vi "质控单元流程步骤.vi"() -> ()   [LabVIEW 2016]
panel:
  out "步骤时间/秒":T1={"步骤1时间"=2, "步骤2时间"=4, "步骤3时间"=2, "步骤4时间"=5, "步骤5时间"=6, "步骤6时间"=3, "步骤7时间"=4, "步骤8时间"=7, "步骤9时间"=8, "步骤10时间"=6}
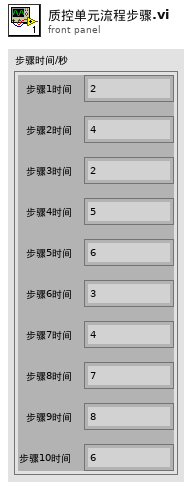
[diagram p1: front panel]
types:
  T1 = cluster{"步骤1时间":i32, "步骤2时间":i32, "步骤3时间":i32, "步骤4时间":i32, "步骤5时间":i32, "步骤6时间":i32, "步骤7时间":i32, "步骤8时间":i32, "步骤9时间":i32, "步骤10时间":i32}
  T2 = enum16{"步骤1", "步骤2", "步骤3", "步骤4", "步骤5", "步骤6", "步骤7", "步骤8", "步骤9", "步骤10"}
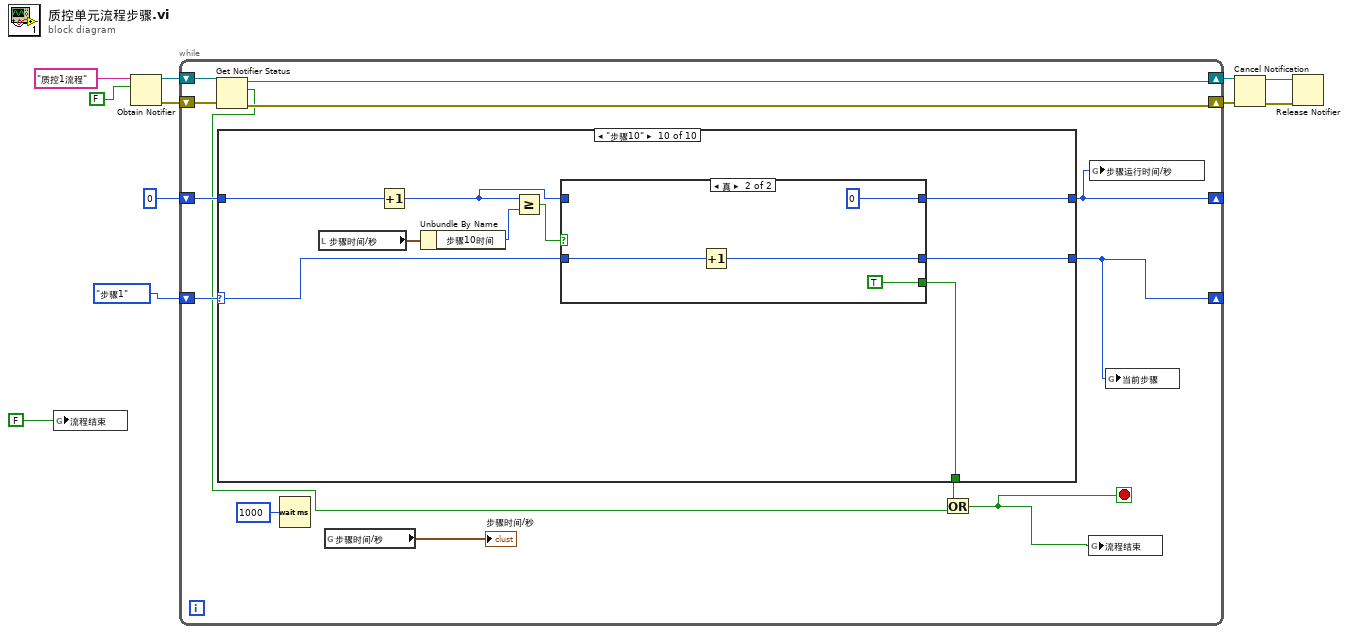
[diagram p0: block diagram]
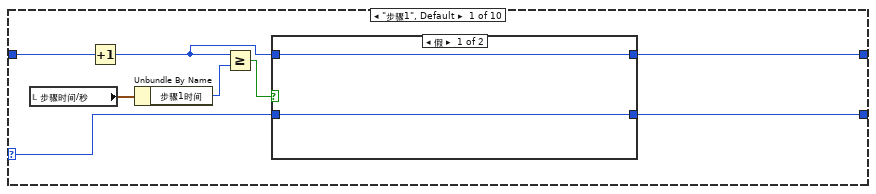
[diagram p2: hidden frame]
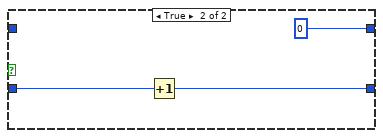
[diagram p3: hidden frame]
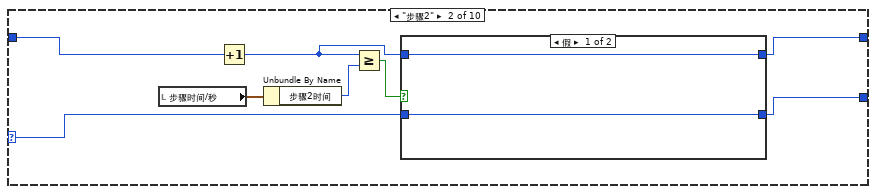
[diagram p4: hidden frame]
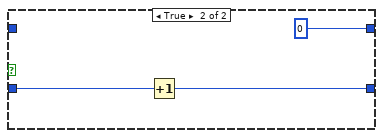
[diagram p5: hidden frame]
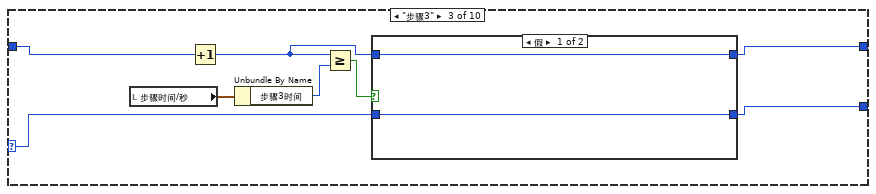
[diagram p6: hidden frame]
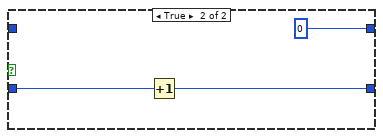
[diagram p7: hidden frame]
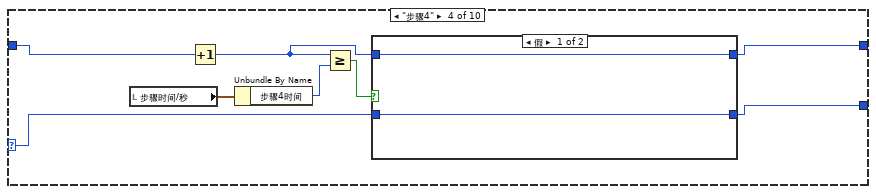
[diagram p8: hidden frame]
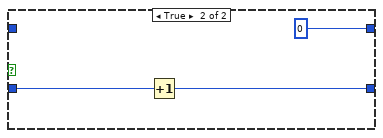
[diagram p9: hidden frame]
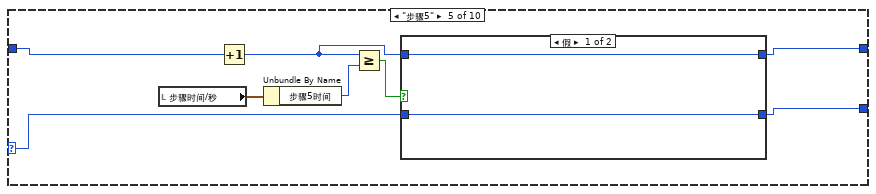
[diagram p10: hidden frame]
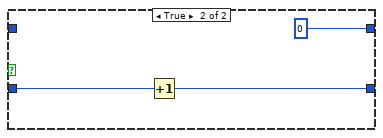
[diagram p11: hidden frame]
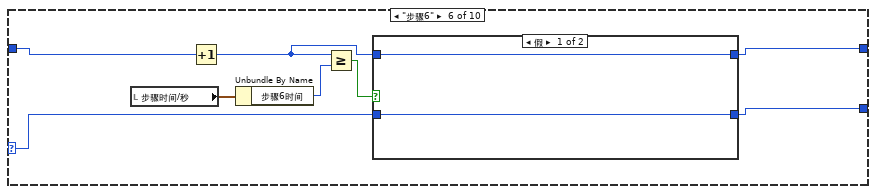
[diagram p12: hidden frame]
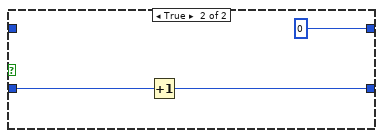
[diagram p13: hidden frame]
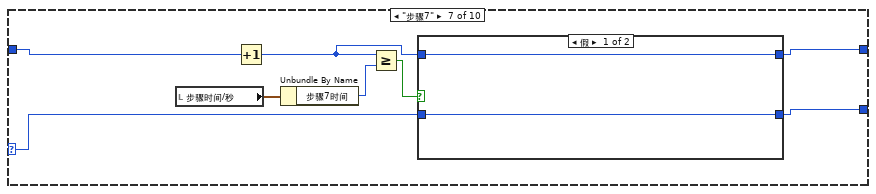
[diagram p14: hidden frame]
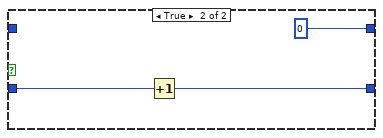
[diagram p15: hidden frame]
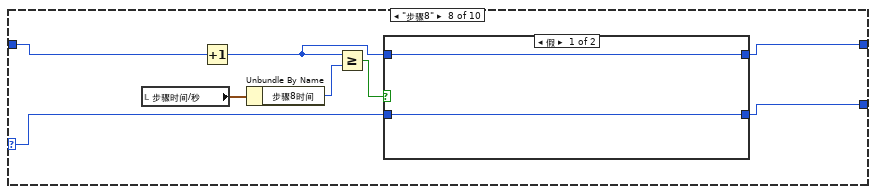
[diagram p16: hidden frame]
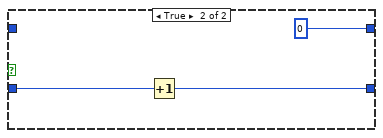
[diagram p17: hidden frame]
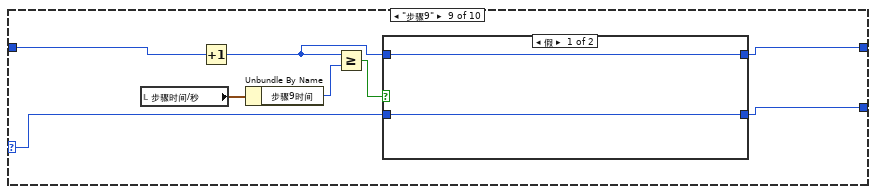
[diagram p18: hidden frame]
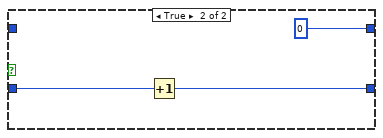
[diagram p19: hidden frame]
diagram:
  n1 = global write "质控单元全局.vi" "流程结束"(FALSE ("流程结束")) -> ()
  n2 = Obtain Notifier(name (unnamed)="质控1流程" ("名称（未命名）"), notification data type=FALSE) -> (notifier out=w7:refnum<notifier>, error out=w6:errorcluster)  [unwired: 2 in, 1 out]
  n3 = while {
    shift-right: [w13] -> _
    shift-left: T2."步骤1" -> [w24]
    shift-right: [w12] -> _
    shift-left: 0 -> [w22]
    shift-right: [w18] -> w3
    shift-left: w7 -> [w20]
    shift-right: [w17] -> w2
    shift-left: w6 -> [w19]
    stop <- w14 stop-if-true
    n4 = Get Notifier Status(notifier=w20, error in (no error)=w19) -> (notifier out=w18:refnum<notifier>, current notification=w16:bool, error out=w17:errorcluster)  [unwired: 2 out]
    n5 = case shown="\"步骤10\"" w24 {
      selector: w24 -> [w26 w40 w53 w66 w79 w92 w105 w118 w131 w145]
      tunnel: [_ _ _ _ _ _ _ _ _ w142] -> w21
      tunnel: w22 -> [w32 w41 w54 w67 w80 w93 w106 w119 w132 w146]
      tunnel: [w28 w39 w52 w65 w78 w91 w104 w117 w130 w144] -> w12
      tunnel: [w25 w38 w51 w64 w77 w90 w103 w116 w129 w143] -> w13
      frame "步骤1", Default {
        n6 = local read "步骤时间/秒"() -> (w31:T1)
        n7 = Increment(x=w32) -> (x+1=w27:i32)
        n8 = Unbundle By Name(w31) -> ("步骤1时间"=w30:i32)
        n9 = Greater Or Equal?(x=w27, y=w30) -> (x >= y?=w29:bool)
        n10 = case shown="假" w29 {
          tunnel: [w34 0] -> w28
          tunnel: w27 -> [w34 _]
          tunnel: w26 -> [w33 w36]
          tunnel: [w33 w35] -> w25
          frame False {
          }
          frame True {
            n11 = Increment(x=w36) -> (x+1=w35:T2)
          }
        }
      }
      frame "步骤2" {
        n12 = local read "步骤时间/秒"() -> (w45:T1)
        n13 = Increment(x=w41) -> (x+1=w42:i32)
        n14 = Unbundle By Name(w45) -> ("步骤2时间"=w44:i32)
        n15 = Greater Or Equal?(x=w42, y=w44) -> (x >= y?=w43:bool)
        n16 = case shown="假" w43 {
          tunnel: [w47 0] -> w39
          tunnel: w42 -> [w47 _]
          tunnel: w40 -> [w46 w49]
          tunnel: [w46 w48] -> w38
          frame False {
          }
          frame True {
            n17 = Increment(x=w49) -> (x+1=w48:T2)
          }
        }
      }
      frame "步骤3" {
        n18 = local read "步骤时间/秒"() -> (w58:T1)
        n19 = Increment(x=w54) -> (x+1=w55:i32)
        n20 = Unbundle By Name(w58) -> ("步骤3时间"=w57:i32)
        n21 = Greater Or Equal?(x=w55, y=w57) -> (x >= y?=w56:bool)
        n22 = case shown="假" w56 {
          tunnel: [w60 0] -> w52
          tunnel: w55 -> [w60 _]
          tunnel: w53 -> [w59 w62]
          tunnel: [w59 w61] -> w51
          frame False {
          }
          frame True {
            n23 = Increment(x=w62) -> (x+1=w61:T2)
          }
        }
      }
      frame "步骤4" {
        n24 = local read "步骤时间/秒"() -> (w71:T1)
        n25 = Increment(x=w67) -> (x+1=w68:i32)
        n26 = Unbundle By Name(w71) -> ("步骤4时间"=w70:i32)
        n27 = Greater Or Equal?(x=w68, y=w70) -> (x >= y?=w69:bool)
        n28 = case shown="假" w69 {
          tunnel: [w73 0] -> w65
          tunnel: w68 -> [w73 _]
          tunnel: w66 -> [w72 w75]
          tunnel: [w72 w74] -> w64
          frame False {
          }
          frame True {
            n29 = Increment(x=w75) -> (x+1=w74:T2)
          }
        }
      }
      frame "步骤5" {
        n30 = local read "步骤时间/秒"() -> (w84:T1)
        n31 = Increment(x=w80) -> (x+1=w81:i32)
        n32 = Unbundle By Name(w84) -> ("步骤5时间"=w83:i32)
        n33 = Greater Or Equal?(x=w81, y=w83) -> (x >= y?=w82:bool)
        n34 = case shown="假" w82 {
          tunnel: [w86 0] -> w78
          tunnel: w81 -> [w86 _]
          tunnel: w79 -> [w85 w88]
          tunnel: [w85 w87] -> w77
          frame False {
          }
          frame True {
            n35 = Increment(x=w88) -> (x+1=w87:T2)
          }
        }
      }
      frame "步骤6" {
        n36 = local read "步骤时间/秒"() -> (w97:T1)
        n37 = Increment(x=w93) -> (x+1=w94:i32)
        n38 = Unbundle By Name(w97) -> ("步骤6时间"=w96:i32)
        n39 = Greater Or Equal?(x=w94, y=w96) -> (x >= y?=w95:bool)
        n40 = case shown="假" w95 {
          tunnel: [w99 0] -> w91
          tunnel: w94 -> [w99 _]
          tunnel: w92 -> [w98 w101]
          tunnel: [w98 w100] -> w90
          frame False {
          }
          frame True {
            n41 = Increment(x=w101) -> (x+1=w100:T2)
          }
        }
      }
      frame "步骤7" {
        n42 = local read "步骤时间/秒"() -> (w110:T1)
        n43 = Increment(x=w106) -> (x+1=w107:i32)
        n44 = Unbundle By Name(w110) -> ("步骤7时间"=w109:i32)
        n45 = Greater Or Equal?(x=w107, y=w109) -> (x >= y?=w108:bool)
        n46 = case shown="假" w108 {
          tunnel: [w112 0] -> w104
          tunnel: w107 -> [w112 _]
          tunnel: w105 -> [w111 w114]
          tunnel: [w111 w113] -> w103
          frame False {
          }
          frame True {
            n47 = Increment(x=w114) -> (x+1=w113:T2)
          }
        }
      }
      frame "步骤8" {
        n48 = local read "步骤时间/秒"() -> (w123:T1)
        n49 = Increment(x=w119) -> (x+1=w120:i32)
        n50 = Unbundle By Name(w123) -> ("步骤8时间"=w122:i32)
        n51 = Greater Or Equal?(x=w120, y=w122) -> (x >= y?=w121:bool)
        n52 = case shown="假" w121 {
          tunnel: [w125 0] -> w117
          tunnel: w120 -> [w125 _]
          tunnel: w118 -> [w124 w127]
          tunnel: [w124 w126] -> w116
          frame False {
          }
          frame True {
            n53 = Increment(x=w127) -> (x+1=w126:T2)
          }
        }
      }
      frame "步骤9" {
        n54 = local read "步骤时间/秒"() -> (w136:T1)
        n55 = Increment(x=w132) -> (x+1=w133:i32)
        n56 = Unbundle By Name(w136) -> ("步骤9时间"=w135:i32)
        n57 = Greater Or Equal?(x=w133, y=w135) -> (x >= y?=w134:bool)
        n58 = case shown="假" w134 {
          tunnel: [w138 0] -> w130
          tunnel: w133 -> [w138 _]
          tunnel: w131 -> [w137 w140]
          tunnel: [w137 w139] -> w129
          frame False {
          }
          frame True {
            n59 = Increment(x=w140) -> (x+1=w139:T2)
          }
        }
      }
      frame "步骤10" {
        n60 = local read "步骤时间/秒"() -> (w150:T1)
        n61 = Increment(x=w146) -> (x+1=w147:i32)
        n62 = Unbundle By Name(w150) -> ("步骤10时间"=w149:i32)
        n63 = Greater Or Equal?(x=w147, y=w149) -> (x >= y?=w148:bool)
        n64 = case shown="真" w148 {
          tunnel: [w152 0] -> w144
          tunnel: w147 -> [w152 _]
          tunnel: w145 -> [w151 w155]
          tunnel: [w151 w154] -> w143
          tunnel: [_ TRUE] -> w142
          frame False {
          }
          frame True {
            n65 = Increment(x=w155) -> (x+1=w154:T2)
          }
        }
      }
    }
    n66 = Wait (ms)(milliseconds to wait=u32 1000 ("等待时间（毫秒）")) -> ()  [unwired: 1 out]
    n67 = global read "质控单元全局.vi" "步骤时间/秒"() -> (→"步骤时间/秒":T1)
    n68 = Or(x=w21, y=w16) -> (x .or. y?=w14:bool)
    n69 = global write "质控单元全局.vi" "流程结束"(w14) -> ()
    n70 = global write "质控单元全局.vi" "步骤运行时间/秒"(w12) -> ()
    n71 = global write "质控单元全局.vi" "当前步骤"(w13) -> ()
  }
  n72 = Cancel Notification(0:w3, 3:w2) -> (8:w5:refnum<notifier>, 11:w4:errorcluster)  [unwired: 1 out]
  n73 = Release Notifier(notifier=w5, error in (no error)=w4) -> ()  [unwired: 1 in, 3 out]
